vi "DACQH.vi"(6 "writeEqualsRead?":bool, 8 "Readback":u32) -> (0 "DACQuWriteTimeout":bool)   [LabVIEW 2014]
uses:
  <vilib>/Platform/TimedLoop/XDataNode/timing_clust.ctl
  <vilib>/Platform/TimedLoop/XDataNode/nitl_modes.ctl
  <vilib>/Platform/TimedLoop/XDataNode/wakeup.ctl
  <vilib>/rvi/Emulation/niFpgaSctlEmulationGetInTimedLoop.vi
  <vilib>/rvi/Emulation/niFpgaEmulationReportErrorSimple.vi
  <vilib>/rvi/Emulation/niFpgaGetClockAttributes.vi
  <vilib>/rvi/Emulation/niFpgaCriticalErrorInLSC.vi
  <vilib>/rvi/interface/RandomDataEmulation/niFpgaRandomDataHandleErrors.vi
  queueHandlerGlobals.vi
  <vilib>/rvi/Emulation/niFpgaProcessEmulError.vi
  <vilib>/Platform/TimedLoop/XDataNode/XDataNode.xnode
  <vilib>/rvi/DataTransferAndStorage/Container/XNode/niFpgaContainer.xnode
  <vilib>/rvi/interface/RandomDataEmulation/nirviRandomDataFpgaReadWriteTemplate.vi
  <vilib>/Platform/TimedLoop/XDataNode/XDNodeRunTimeDep.lvlib
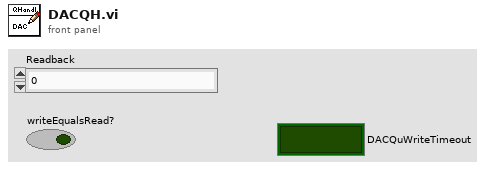
[diagram p1: front panel]
types:
  T1 = typedef "XDNodeRunTimeDep.lvlib/timing_clust.ctl" = cluster{"Expected End [f-1]":u64, "Actual End [f-1]":u64, "Finished Late? [f-1]":bool, "Expected End [i-1]":u64, "Actual End [i-1]":u64, "Finished Late? [i-1]":bool, "Expected Start [i]":u64, "Actual Start [i]":u64, "Expected Start [f]":u64, "Actual Start [f]":u64, "Source Name":string, "Structure Name":string, "Period":i64, "Deadline":i64, "Offset":i64, "Start":i64, "Priority":i32, "Timeout":i32, "Mode":T2, "Wakeup Reason":T3, "Error":errorcluster, "Source Type":string, "Secondary Source Type":string, "Global End Time":u64, "Global Start Time":u64, "Frame Duration":u64, "Iteration Duration":u64, "Assigned CPU":i32, "I/O Scan Engine Mode":u32}
  T2 = typedef "XDNodeRunTimeDep.lvlib/nitl_modes.ctl" = enum32{"No Change", "Process missed periods, maintain original phase", "Discard missed periods, maintain original phase", "Process missed periods, ignore original phase", "Discard missed periods, ignore original phase"}
  T3 = typedef "XDNodeRunTimeDep.lvlib/wakeup.ctl" = enum32{"Normal", "Aborted", "Asynchronous wakeup", "Timing source error", "Timed loop error", "Timeout"}
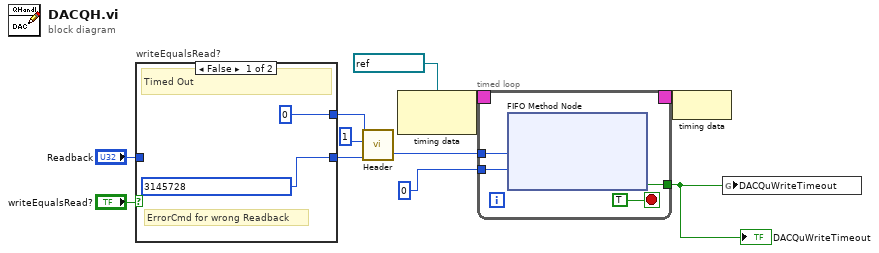
[diagram p0: block diagram]
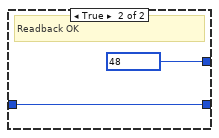
[diagram p2: hidden frame]
diagram:
  n1 = case "writeEqualsRead?" shown="False" "writeEqualsRead?" {
    tunnel: [u8 0 ("8BitHead") u8 48 ("8BitHead")] -> w11
    tunnel: "Readback" -> [_ w14]
    tunnel: [u32 3145728 ("Readback") w14] -> w7
    frame False {
      # "ErrorCmd for wrong Readback"
      # "Timed Out"
    }
    frame True {
      # "Readback OK"
    }
  }
  n2 = call "Header.vi"("23BitData"=w7, "1BitHeaderIndex"=u8 1, "8BitHead"=w11) -> ("32BitOutput"=w9:u32)  [unwired: 2 in]
  n3 = node-c288(refnum<k21> "100MHz" ("Source Name")) -> (w3:T1)
  n4 = timed-loop {
    timing: w3 -> [_]
    timing-out: [_] -> w2
    tunnel: w9 -> [w19]
    tunnel: 0 ("Timeout") -> [w18]
    tunnel: [w17] -> w4
    stop <- TRUE stop-if-true
    n5 = xnode ("FIFO Method Node")("Element"=w19, "Timeout"=w18) -> ("Timed Out?"=w17:bool)  [unwired: 1 in, 1 out]
  }
  "DACQuWriteTimeout" <- w4
  n6 = node-c288(w2) -> ()
  n7 = global write "queueHandlerGlobals.vi" "DACQuWriteTimeout"(w4) -> ()
